vi "endValueChange.vi"(8 "error in (no error)":errorcluster, 9 "oldValue":dbl, 10 "newValue":dbl, 11 "ScanCreator in":refnum<class "ScanCreator.lvclass">) -> (0 "error out":errorcluster, 3 "ScanCreator out":refnum<class "ScanCreator.lvclass">)   [LabVIEW 2011, in "Views.lvlib" / "ScriptEditor.lvlib" / "ScanCreator.lvclass"]
uses:
  ScanCreator.lvclass
  ScanCreator.lvclass/ScanCreator.ctl
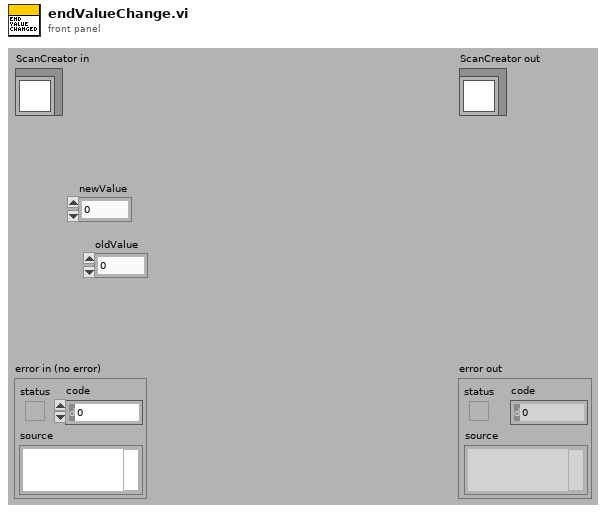
[diagram p1: front panel]
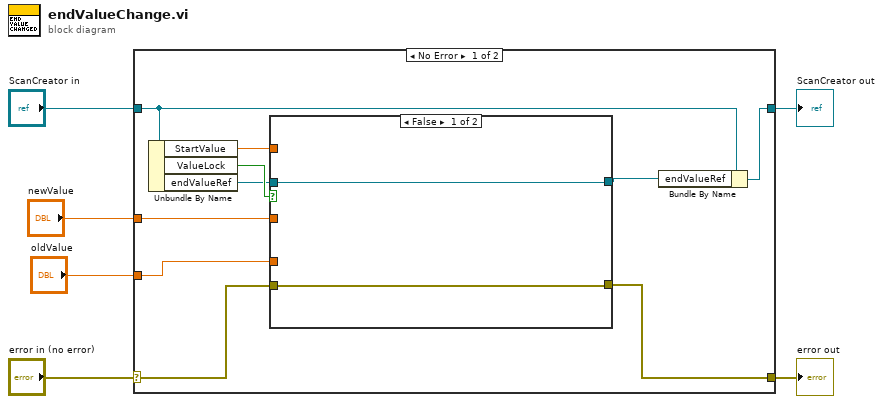
[diagram p0: block diagram]
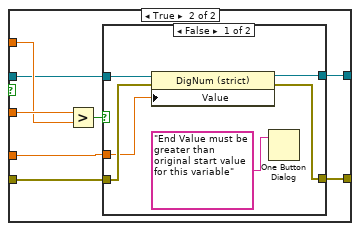
[diagram p2: hidden frame]
diagram:
  n1 = case shown="No Error" "error in (no error)" {
    selector: "error in (no error)" -> [w11 w36]
    tunnel: [w10 w36] -> w5
    tunnel: [w7 w35] -> w3
    tunnel: "ScanCreator in" -> [w8 w35]
    tunnel: "newValue" -> [w13 _]
    tunnel: "oldValue" -> [w12 _]
    frame No Error {
      n2 = Unbundle By Name(w8) -> ("StartValue"=w15:dbl, "ValueLock"=w16:bool, "endValueRef"=w14:refnum<vi>)
      n3 = case shown="False" w16 {
        tunnel: w11 -> [w17 w21]
        tunnel: w15 -> [_ w25]
        tunnel: w14 -> [w18 w22]
        tunnel: w13 -> [_ w26]
        tunnel: w12 -> [_ w23]
        tunnel: [w18 w20] -> w9
        tunnel: [w17 w19] -> w10
        frame False {
        }
        frame True {
          n4 = Greater?(x=w26, y=w25) -> (0:w24:bool)
          n5 = case shown="False" w24 {
            tunnel: w23 -> [w30 _]
            tunnel: w22 -> [w32 w34]
            tunnel: w21 -> [w31 w33]
            tunnel: [w29 w34] -> w20
            tunnel: [w28 w33] -> w19
            frame False {
              n6 = property class="DigNum (strict)"(reference=w32, error in=w31, "Value"=w30) -> (reference out=w29:refnum<vi>, error out=w28:errorcluster)
              n7 = One Button Dialog(message="End Value must be greater than original start value for this variable") -> ()  [unwired: 1 in, 1 out]
            }
            frame True {
            }
          }
        }
      }
      n8 = Bundle By Name(cluster=w8, "endValueRef"=w9) -> (w7:refnum<class "ScanCreator.lvclass">)
    }
    frame Error {
    }
  }
  "error out" <- w5
  "ScanCreator out" <- w3
